vi "Get main page properties.vi"(8 "error in":errorcluster, 11 "Item Ref in":T2 format="%.0x") -> (0 "error out":errorcluster, 2 "main page properties":T1, 3 "Item Ref out":T2 format="%.0x")   [LabVIEW 2019, in "HLA Custom Device System Explorer.lvlib"]
uses:
  HLA Custom Device System Explorer.lvlib
  <vilib>/NI VeriStand/Custom Device API/Custom Device Item Ref.ctl
  Shared/main_page_config.ctl
  Shared/Constants.vi
  <vilib>/NI VeriStand/Custom Device API/Get Item Property (String).vi
  <vilib>/NI VeriStand/Custom Device API/Get Item Property (Path).vi
  <vilib>/NI VeriStand/Custom Device API/Custom Device API.lvlib
  Shared/HLA Custom Device Shared.lvlib
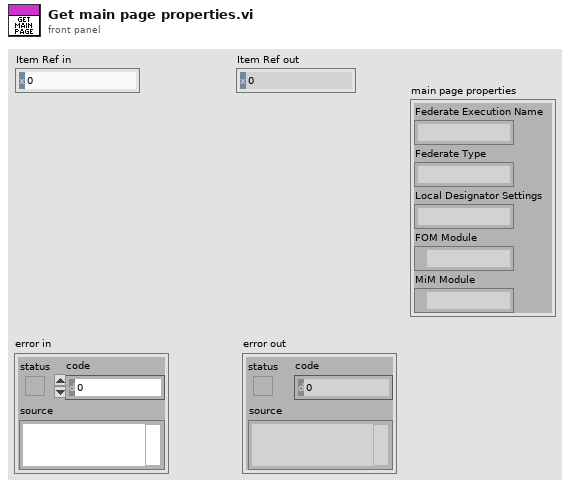
[diagram p1: front panel]
types:
  T1 = typedef "HLA Custom Device Shared.lvlib/main_page_config.ctl" = cluster{"Federate Execution Name":string, "Federate Type":string, "Local Designator Settings":string, "FOM Module":path, "MiM Module":path}
  T2 = typedef "Custom Device API.lvlib/Custom Device Item Ref.ctl" = u64
  T3 = cluster{"Value":string, "Value":string, "Value":string, "Value":path, "Value":path}
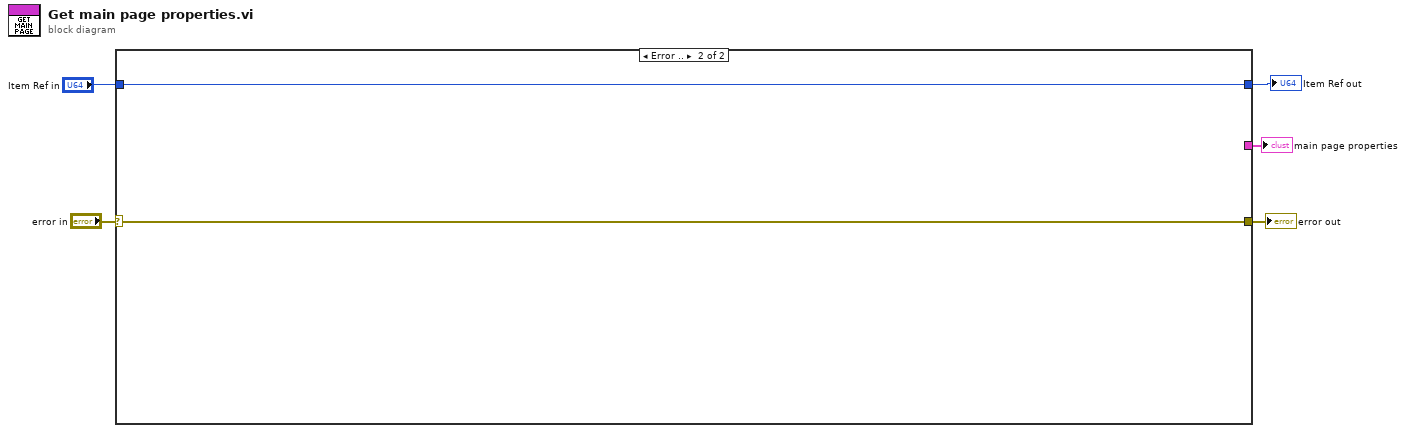
[diagram p0: block diagram]
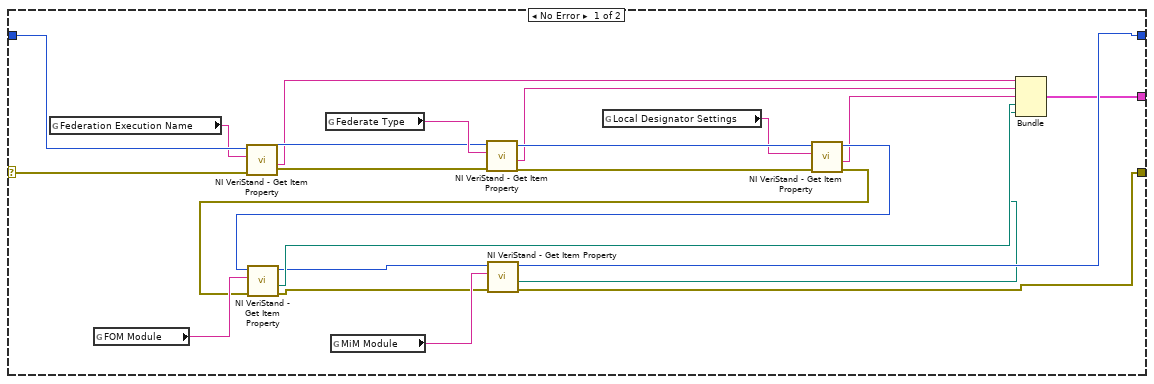
[diagram p2: hidden frame]
diagram:
  n1 = case shown="Error .." "error in" {
    selector: "error in" -> [w27 w29]
    tunnel: [w15 w29] -> w4
    tunnel: [w14 w30] -> w3
    tunnel: "Item Ref in" -> [w28 w30]
    tunnel: [w6 _] -> w1
    frame No Error {
      n2 = global read "Constants.vi" "Federation Execution Name"() -> (w26:string)
      n3 = global read "Constants.vi" "FOM Module"() -> (w23:string)
      n4 = call-poly <vilib>:"NI VeriStand - Get Item Property.vi"("error in (no error)"=w27, "Property Name"=w26, "Item Ref in"=w28) -> ("error out"=w21:errorcluster, "Value"=w13:string, "Item Ref out"=w22:T2)  [unwired: 5 in, 1 out]
      n5 = global read "Constants.vi" "Federate Type"() -> (w25:string)
      n6 = global read "Constants.vi" "MiM Module"() -> (w24:string)
      n7 = call-poly <vilib>:"NI VeriStand - Get Item Property.vi"("error in (no error)"=w21, "Property Name"=w25, "Item Ref in"=w22) -> ("error out"=w19:errorcluster, "Value"=w12:string, "Item Ref out"=w20:T2)  [unwired: 5 in, 1 out]
      n8 = global read "Constants.vi" "Local Designator Settings"() -> (w11:string)
      n9 = call-poly <vilib>:"NI VeriStand - Get Item Property.vi"("error in (no error)"=w19, "Property Name"=w11, "Item Ref in"=w20) -> ("error out"=w17:errorcluster, "Value"=w10:string, "Item Ref out"=w18:T2)  [unwired: 5 in, 1 out]
      n10 = call-poly <vilib>:"NI VeriStand - Get Item Property.vi"("error in (no error)"=w17, "Property Name"=w23, "Item Ref in"=w18) -> ("error out"=w16:errorcluster, "Value"=w9:path, "Item Ref out"=w8:T2)  [unwired: 5 in, 1 out]
      n11 = call-poly <vilib>:"NI VeriStand - Get Item Property.vi"("error in (no error)"=w16, "Property Name"=w24, "Item Ref in"=w8) -> ("error out"=w15:errorcluster, "Value"=w7:path, "Item Ref out"=w14:T2)  [unwired: 5 in, 1 out]
      n12 = Bundle("Value"=w13, "Value"=w12, "Value"=w10, "Value"=w9, "Value"=w7) -> (w6:T3)  [unwired: 1 in]
    }
    frame Error {
    }
  }
  "error out" <- w4
  "Item Ref out" <- w3
  "main page properties" <- w1
